vi "setFullScales.vi"(8 "error out 2":errorcluster, 11 "Protocol_Generic out 2":refnum<class "Protocol_Logging.lvclass">) -> (0 "error out":errorcluster, 3 "Protocol_Generic out":refnum<class "Protocol_Logging.lvclass">)   [LabVIEW 2011, in "Protocol_Logging.lvclass"]
uses:
  Protocol_Logging.lvclass
  Protocol_Logging.lvclass/Protocol_Logging.ctl
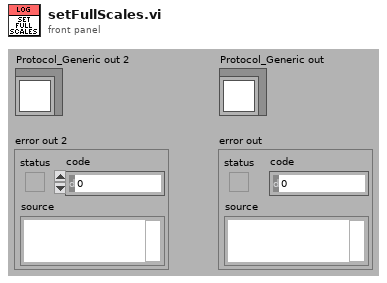
[diagram p1: front panel]
types:
  T1 = cluster{"Axis Information":cluster{"Device ID":i32, "Device Name":string, "Device Type":i32}[], "Axis Selector":i32[], "Control Modes out":u16[], "error out":errorcluster, "Channel Data":cluster{"Name":string, "Type":i32, "SI Full Scale":dbl, "Full Scale":dbl, "Units String":string, "Display Format":string, "Gauge Length":dbl}[][]}
  T2 = cluster{"Name":string, "Type":i32, "SI Full Scale":dbl, "Full Scale":dbl, "Units String":string, "Display Format":string, "Gauge Length":dbl}[][]
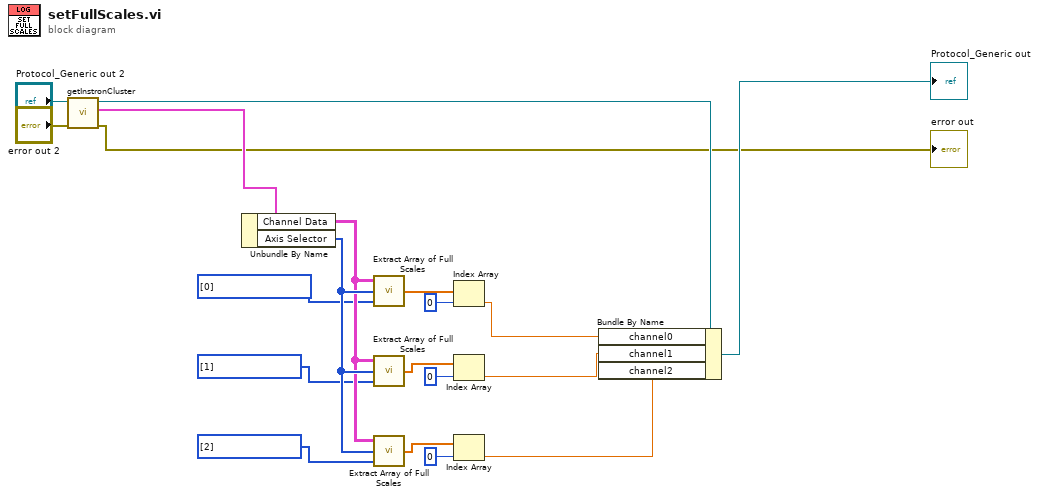
[diagram p0: block diagram]
diagram:
  w6 = u16[] [2] items=["Channel 1", "Channel 2", "Channel 3", "Channel 4"] ("Channel")
  w5 = u16[] [1] items=["Channel 1", "Channel 2", "Channel 3", "Channel 4"] ("Channel")
  w4 = u16[] [0] items=["Channel 1", "Channel 2", "Channel 3", "Channel 4"] ("Channel")
  n1 = call-dynamic "getInstronCluster.vi"("error in (no error)"="error out 2", "Protocol_Generic in"="Protocol_Generic out 2") -> ("error out"=→"error out":errorcluster, "InstronCluster"=w13:T1, "Protocol_Generic out"=w16:refnum<class "Protocol_Logging.lvclass">)  [unwired: 7 in]
  n2 = Unbundle By Name(w13) -> ("Channel Data"=w14:T2, "Axis Selector"=w15:i32[])
  n3 = call "Extract Array of Full Scales.vi"("Channel"=w4, "Axis Selector"=w15, "Axis\nChannel"=w14) -> ("Full Scales"=w7:dbl[])
  n4 = call "Extract Array of Full Scales.vi"("Channel"=w5, "Axis Selector"=w15, "Axis\nChannel"=w14) -> ("Full Scales"=w12:dbl[])
  n5 = call "Extract Array of Full Scales.vi"("Channel"=w6, "Axis Selector"=w15, "Axis\nChannel"=w14) -> ("Full Scales"=w11:dbl[])
  n6 = Index Array(array=w7, index=0) -> (element=w18:dbl)
  n7 = Index Array(array=w12, index=0) -> (element=w19:dbl)
  n8 = Index Array(array=w11, index=0) -> (element=w20:dbl)
  n9 = Bundle By Name(cluster=w16, "channel0"=w18, "channel1"=w19, "channel2"=w20) -> (→"Protocol_Generic out":refnum<class "Protocol_Logging.lvclass">)
